vi "PID.vi"() -> ()   [LabVIEW 2016]
panel:
  out "ControlValues":sgl[](array[numeric])
  in  "MeasuredValues":sgl[](array[numeric])=[0.0, 0.0, 0.0, 0.0, 0.0, 0.0, 0.0, 0.0, 0.0, 0.0, 0.0, 0.0, 0.0, 0.0, 0.0, 0.0, 0.0, 0.0, 0.0, 0.0, 0.0, 0.0, 0.0, 0.0, 0.0, 0.0, 0.0, 0.0, 0.0, 0.0, 0.0, 0.0, 0.0, 0.0, 0.0, 0.0]
  in  "Setpoints":sgl[](array[numeric])=[0.0, 0.0, 0.0, 0.0, 0.0, 0.0, 0.0, 0.0, 0.0, 0.0, 0.0, 0.0, 0.0, 0.0, 0.0, 0.0, 0.0, 0.0, 0.0, 0.0, 0.0, 0.0, 0.0, 0.0, 0.0, 0.0, 0.0, 0.0, 0.0, 0.0, 0.0, 0.0, 0.0, 0.0, 0.0, 0.0]
  out "C":sgl
  out "B":sgl
  out "A":sgl
  in  "Kd":sgl
  in  "Ki":sgl
  in  "Kp":sgl
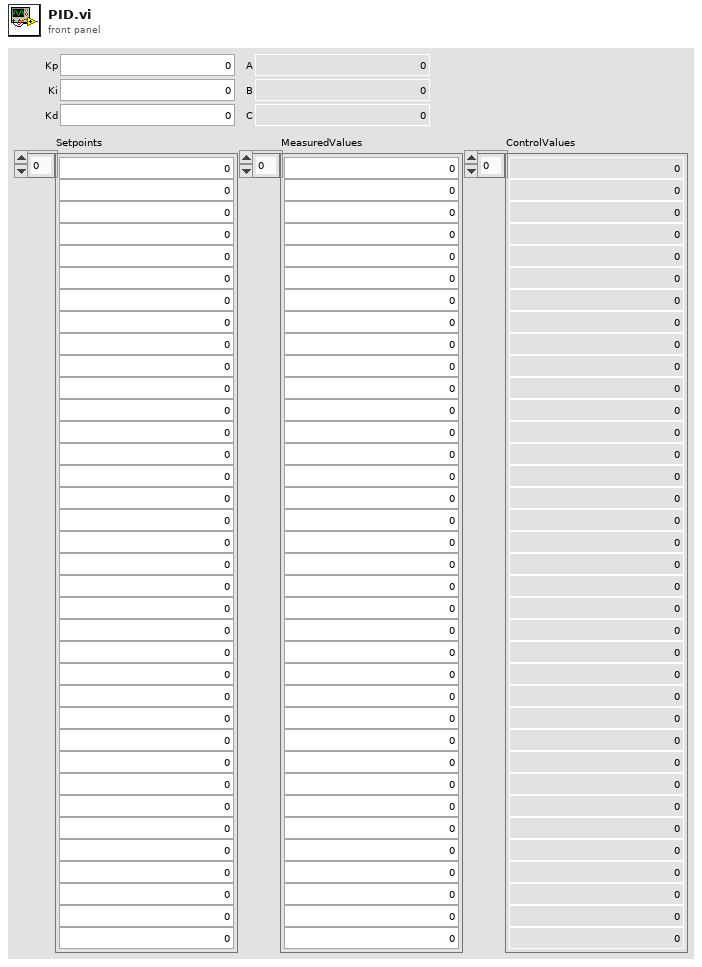
[diagram p1: front panel]
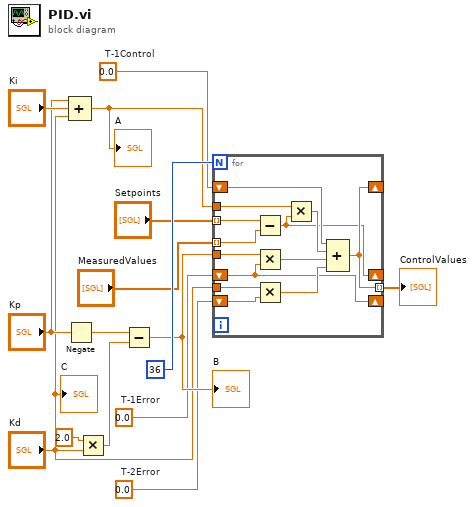
[diagram p0: block diagram]
diagram:
  w2 = sgl 0.0  # T-1Control
  w3 = sgl 0.0  # T-2Error
  w4 = sgl 0.0  # T-1Error
  n1 = Negate(x="Kp") -> (-x=w13:sgl)
  n2 = Compound Arithmetic op=ADD("Kp", "Ki", "Kd") -> (w9:sgl)
  "A" <- w9
  n3 = Multiply(x=sgl 2.0, y="Kd") -> (x*y=w11:sgl)
  n4 = Subtract(x=w13, y=w11) -> (x-y=w8:sgl)
  "B" <- w8
  n5 = for {
    N: 36 -> [_]
    tunnel: w9 -> [w25]
    tunnel: w8 -> [w24]
    tunnel: "Kd" -> [w23]
    tunnel: "Setpoints" -> [w28] mode=indexing
    tunnel: "MeasuredValues" -> [w27] mode=indexing
    shift-right: [w17] -> _
    shift-left: w4 -> [w16]
    shift-right: [w16] -> _
    shift-left: w3 -> [w18]
    shift-right: [w19] -> _
    shift-left: w2 -> [w26]
    tunnel: [w19] -> w1 mode=indexing
    n6 = Subtract(x=w28, y=w27) -> (x-y=w17:sgl)
    n7 = Multiply(x=w24, y=w16) -> (x*y=w21:sgl)
    n8 = Multiply(x=w23, y=w18) -> (x*y=w20:sgl)
    n9 = Multiply(x=w25, y=w17) -> (x*y=w22:sgl)
    n10 = Compound Arithmetic op=ADD(w26, w22, w21, w20) -> (w19:sgl)
  }
  "ControlValues" <- w1
  "C" <- "Kd"
